vi "CreateGraphics.vi"(8 "error in (no error)":errorcluster, 11 "LcPictureBox in":refnum<class "LcPictureBox.lvclass">) -> (0 "error out":errorcluster, 2 "CreateGraphics":refnum<k24>, 3 "LcPictureBox out":refnum<class "LcPictureBox.lvclass">)   [LabVIEW 2020, in "LcPictureBox.lvclass"]
uses:
  LcPictureBox.lvclass
  System.Windows.Forms
  System.Drawing
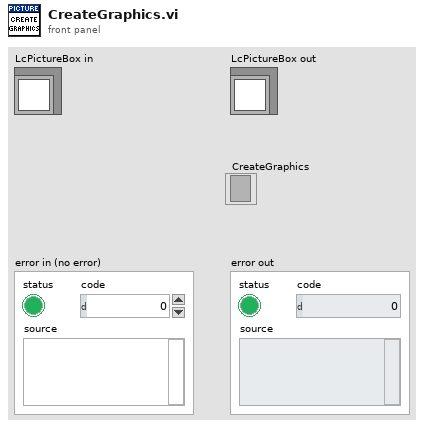
[diagram p1: front panel]
types:
  T1 = typedef "LcPictureBox.lvclass/ObjectAttributes.ctl" = cluster{"PictureBox":refnum<k24>, "ImageSize":cluster{"Width":i32, "Height":i32}, "PenMemory":map{cluster{"Alpha(100%)":dbl, "Color(Black)":u32, "Pen(Width=1, Solid)":T2}, refnum<k24>}, "GraphicsRef":refnum<k24>, "BrushMemory":map{cluster{"Alpha(100%)":dbl, "Color(Black)":u32}, refnum<k24>}, "Images":refnum<k24>[], "ImageIndex":i32, "BgColor(None)":u32, "LoadedImages":map{string, cluster{"ImageOut":refnum<k24>, "ImageSize":cluster{"Width":i32, "Height":i32}}}, "ColorsMemory":map{cluster{"Alpha(100%)":dbl, "Color(Black)":u32}, refnum<k24>}, "CacheSize":i32, "PictureBoxActiveXReference":refnum<vi>, "Scale":sgl, "Offset":cluster{"x":sgl, "y":sgl}, "zoom_center":cluster{"X":i32, "Y":i32}, "ImagesCreated":refnum<k24>[]}
  T2 = typedef "LcPictureBox.lvclass/Pen.ctl" = cluster{"Width":u16, "Style":enum32{"Solid", "Dash", "Dot", "DashDot", "DashDotDot"}}
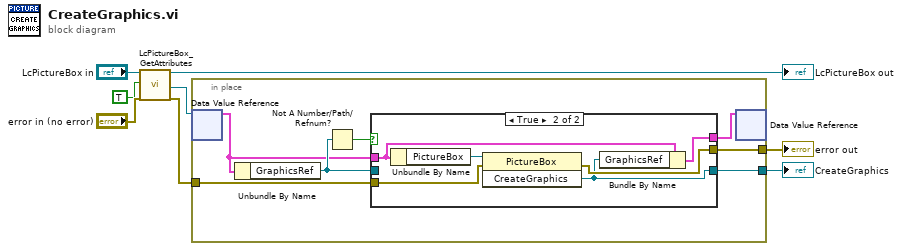
[diagram p0: block diagram]
diagram:
  n1 = call "LcPictureBox_GetAttributes.vi"("reference in"="LcPictureBox in", "OnlyGetDvrReference(False)"=TRUE, "error in (no error)"="error in (no error)") -> ("reference out"=→"LcPictureBox out":refnum<class "LcPictureBox.lvclass">, "DataRef"=w4:refnum<data-value>, "error out"=w3:errorcluster)  [unwired: 13 in, 1 out]
  n2 = in-place {
    in-place-border: w3 -> [w14]
    in-place-border: [w13] -> w2
    in-place-border: [w12] -> w1
    n3 = in-place-dvr #1(w4) -> (w9:T1)  [unwired: 1 out]
    n4 = Unbundle By Name(w9) -> ("GraphicsRef"=w11:refnum<k24>)
    n5 = Not A Number/Path/Refnum?(number/path/refnum=w11) -> (NaN/Path/Refnum?=w15:bool)
    n6 = case shown="True" w15 {
      tunnel: w14 -> [w17 w24]
      tunnel: [w17 w23] -> w13
      tunnel: [w18 w21] -> w12
      tunnel: w11 -> [w18 _]
      tunnel: w9 -> [w16 w20]
      tunnel: [w16 w22] -> w10
      frame False {
      }
      frame True {
        n7 = Unbundle By Name(w20) -> ("PictureBox"=w19:refnum<k24>)
        n8 = invoke class="PictureBox" method="CreateGraphics"(reference=w19, error in=w24) -> (error out=w23:errorcluster, "CreateGraphics"=w21:refnum<k24>)  [unwired: 1 in, 1 out]
        n9 = Bundle By Name(cluster=w20, "GraphicsRef"=w21) -> (w22:T1)
      }
    }
    n10 = in-place-dvr #1(w10) -> ()  [unwired: 2 out]
  }
  "error out" <- w2
  "CreateGraphics" <- w1
